vi "Binary to One Hot (I32).vi"(7 "Binary Number":u32 format="%032b") -> (8 "One Hot Encoded Number":u32 format="%032b")   [LabVIEW 2010]
doc: "This code converts Binary U8 to One hot Encoded Number version of leading one detector from MSB.\n\n000011110000 -- input\n111100001111 -- invert\n111100010000 -- add 1\n000000010000 -- and with input.\n\nexample 2:\n1010101011 -- input\n0101010100 -- invert\n0101010101 -- add 1\n0000000001 -- and with input"
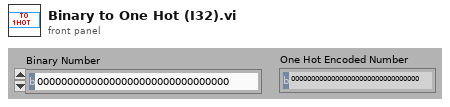
[diagram p1: front panel]
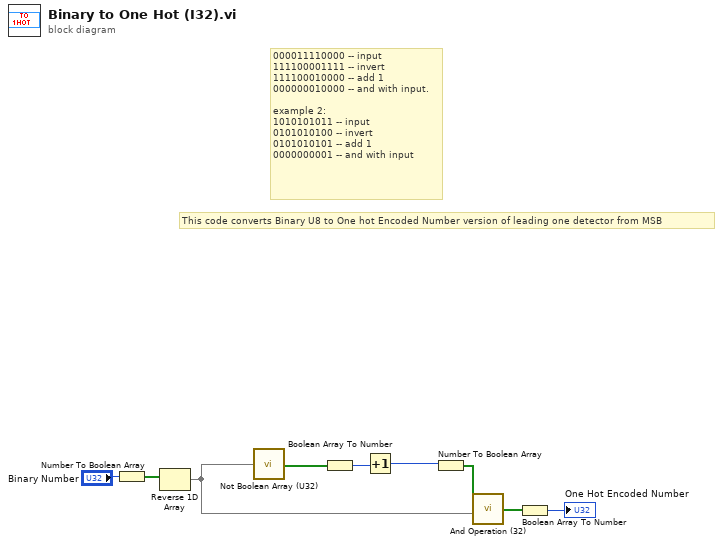
[diagram p0: block diagram]
diagram:
  # "This code converts Binary U8 to One hot Encoded Number version of leading one detector from MSB"
  # "000011110000 -- input\n111100001111 -- invert\n111100010000 -- add 1\n000000010000 -- and with input.\n\nexample 2:\n1010101011 -- input\n0101010100 -- invert\n0101010101 -- add 1\n0000000001 -- and with input"
  n1 = Number To Boolean Array(number="Binary Number") -> (Boolean array=w5:bool[])
  n2 = Reverse 1D Array(array=w5) -> (reversed array=w1:bool[])
  n3 = call "Not Boolean Array (U32).vi"("X"=w1) -> ("Not X"=w2:bool[])  [unwired: 4 in]
  n4 = Boolean Array To Number(Boolean array=w2) -> (number=w9:u32)
  n5 = Increment(x=w9) -> (x+1=w7:u32)
  n6 = Number To Boolean Array(number=w7) -> (Boolean array=w6:bool[])
  n7 = call "And Operation (32).vi"("X"=w6, "Y"=w1) -> ("X.and.Y?"=w4:bool[])  [unwired: 5 in]
  n8 = Boolean Array To Number(Boolean array=w4) -> (number=→"One Hot Encoded Number":u32)
